vi "MHM Get Interface Info.vi"(8 "error in (no error)":errorcluster, 10 "ulIndex":u32, 11 "ulMHMHandle":u32) -> (0 "error out":errorcluster, 2 "pcInterfaceInfo":string, 3 "function return":u32)   [LabVIEW 2017, in "MHM_1SL_interface.lvlib"]
uses:
  MHM_1SL_interface.lvlib
  SSI_Tool/DUT_Interface/lv_interface/lib/MHM_1SL_interface.dll
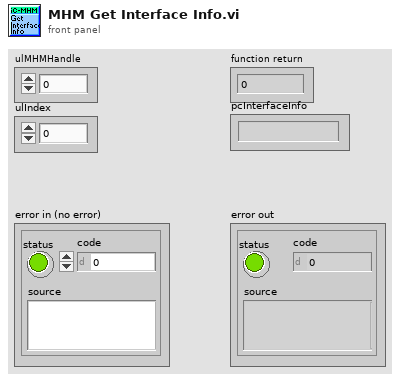
[diagram p1: front panel]
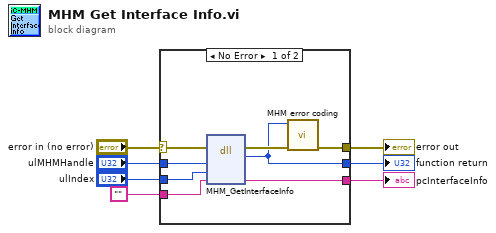
[diagram p0: block diagram]
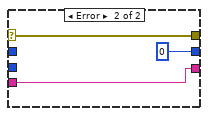
[diagram p2: hidden frame]
diagram:
  n1 = case shown="No Error" "error in (no error)" {
    selector: "error in (no error)" -> [w15 w17]
    tunnel: "ulMHMHandle" -> [w14 _]
    tunnel: [w12 w17] -> w5
    tunnel: [w11 u32 0] -> w4
    tunnel: [w10 w16] -> w3
    tunnel: "ulIndex" -> [w9 _]
    tunnel: "" -> [w8 w16]
    frame No Error {
      n2 = dll-call lib="C:/workspace/project/scancon/sw/SSI_Tool/DUT_Interface/lv_interface/lib/MHM_1SL_interface.dll" fn="MHM_GetInterfaceInfo"(error in=w15, "ulMHMHandle"=w14, "ulIndex"=w9, "pcInterfaceInfo"=w8) -> (error out=w13:errorcluster, "return type"=w11:u32, "pcInterfaceInfo"=w10:string)  [unwired: 4 in, 1 out]
      n3 = call "MHM error coding.vi"("error in (no error)"=w13, "function return in"=w11) -> ("error out"=w12:errorcluster)  [unwired: 9 in]
    }
    frame Error {
    }
  }
  "function return" <- w4
  "error out" <- w5
  "pcInterfaceInfo" <- w3
